vi "Bundle Command.vi"(8 "error in (no error)":errorcluster, 9 "command":T1=enum."Rx", 10 "command parameters":T2, 11 "Plugin Thread in":refnum<class "Plugin Thread.lvclass">) -> (0 "error out":errorcluster, 2 "command":T3={"Command"=enum."Rx", "Parameters"={"arg1"=0, "arg2"=0}}, 3 "Plugin Thread out":refnum<class "Plugin Thread.lvclass">)   [LabVIEW 2017, in "DSF Core.lvlib" / "Plugin Thread.lvclass"]
uses:
  Thread/Plugin/Plugin Thread.lvclass
  Interfaces/Transceiver Interface/Command Data.ctl
  Interfaces/Transceiver Interface/Command.ctl
  Interfaces/Transceiver Interface/Command Parameters.ctl
  Interfaces/Transceiver Interface/Plugin Interface.lvclass
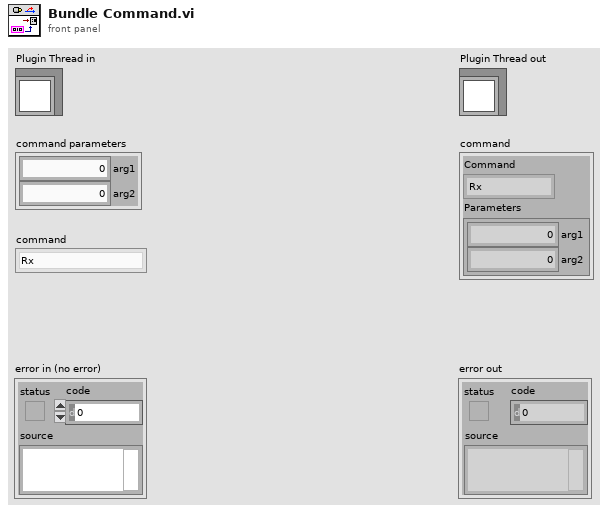
[diagram p1: front panel]
types:
  T1 = typedef "DSF Core.lvlib/Plugin Interface.lvclass/Command.ctl" = enum8{"Set Inline Buffer", "Rx", "Tx", "Shutdown"}
  T2 = typedef "DSF Core.lvlib/Plugin Interface.lvclass/Command Parameters.ctl" = cluster{"arg1":u64, "arg2":u64}
  T3 = typedef "DSF Core.lvlib/Plugin Interface.lvclass/Command Data.ctl" = cluster{"Command":T1, "Parameters":T2}
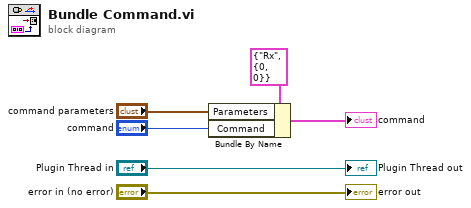
[diagram p0: block diagram]
diagram:
  n1 = Bundle By Name(cluster=T3 {"Command"=enum."Rx", "Parameters"={"arg1"=0, "arg2"=0}} ("command"), "Parameters"="command parameters", "Command"="command") -> (→"command":T3)
  "error out" <- "error in (no error)"
  "Plugin Thread out" <- "Plugin Thread in"
